vi "ConfigureDataEventProperties.vi"(11 "operating state":T2) -> (3 "Sweep Param":T1)   [LabVIEW 2017, in "EmsaDataEventCreator.lvlib"]
uses:
  <vilib>/addons/InsightCM/Devices/Shared/Emsa/EmsaDataEventCreator/EmsaDataEventCreator.lvlib
  <vilib>/addons/InsightCM/MessageBus/Base/controls/OperatingState.ctl
  <vilib>/addons/InsightCM/MessageBus/Base/controls/KeyValuePair.ctl
  <vilib>/addons/InsightCM/MessageBus/Base/controls/Trigger.ctl
  <vilib>/addons/InsightCM/MessageBus/Base/controls/Condition.ctl
  <vilib>/addons/InsightCM/Devices/Shared/Emsa/EmsaDataEventCreator/controls/SweepParams.ctl
  <vilib>/addons/InsightCM/Utilities/PropertyHelpers/PropertyHelpers.lvlib
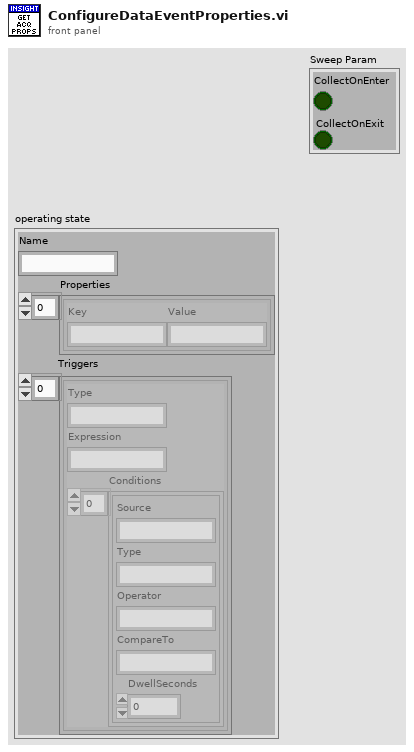
[diagram p1: front panel]
types:
  T1 = typedef "EmsaDataEventCreator.lvlib/SweepParams.ctl" = cluster{"CollectOnEnter":bool, "CollectOnExit":bool}
  T2 = typedef "OperatingState.ctl" = cluster{"Name":string, "Properties":T3[], "Triggers":T4[]}
  T3 = typedef "KeyValuePair.ctl" = cluster{"Key":string, "Value":string}
  T4 = typedef "Trigger.ctl" = cluster{"Type":string, "Expression":string, "Conditions":T5[]}
  T5 = typedef "Condition.ctl" = cluster{"Source":string, "Type":string, "Operator":string, "CompareTo":string, "DwellSeconds":dbl}
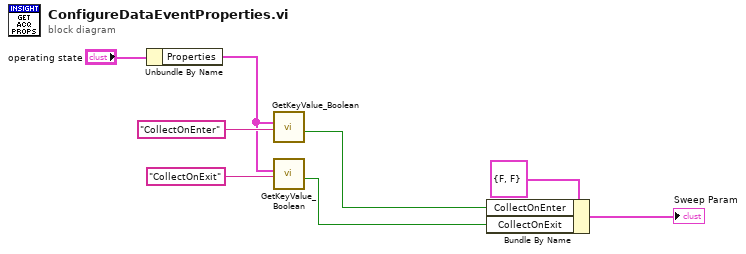
[diagram p0: block diagram]
diagram:
  n1 = Unbundle By Name("operating state") -> ("Properties"=w5:T3[])
  n2 = call <vilib>:"GetKeyValue_Boolean.vi"("key"="CollectOnEnter", "key value pairs"=w5) -> ("value"=w3:bool)  [unwired: 7 in, 2 out]
  n3 = call <vilib>:"GetKeyValue_Boolean.vi"("key"="CollectOnExit", "key value pairs"=w5) -> ("value"=w2:bool)  [unwired: 7 in, 2 out]
  n4 = Bundle By Name(cluster=T1 {"CollectOnEnter"=FALSE, "CollectOnExit"=FALSE} ("AcqParams"), "CollectOnEnter"=w3, "CollectOnExit"=w2) -> (→"Sweep Param":T1)
